vi "Send Message.vi"(6 "Reply to...":refnum<class "Send.lvclass">, 8 "error in (no error)":errorcluster, 10 "Message":refnum<class "MSG.lvclass">, 11 "MSR Parent in":refnum<class "Send.lvclass">) -> (0 "error out":errorcluster, 3 "MSR Parent out":refnum<class "Send.lvclass">)   [LabVIEW 2011, in "Messenging.lvlib" / "Send.lvclass"]
uses:
  Send.lvclass
  TextVarientMessage/MSG.lvclass
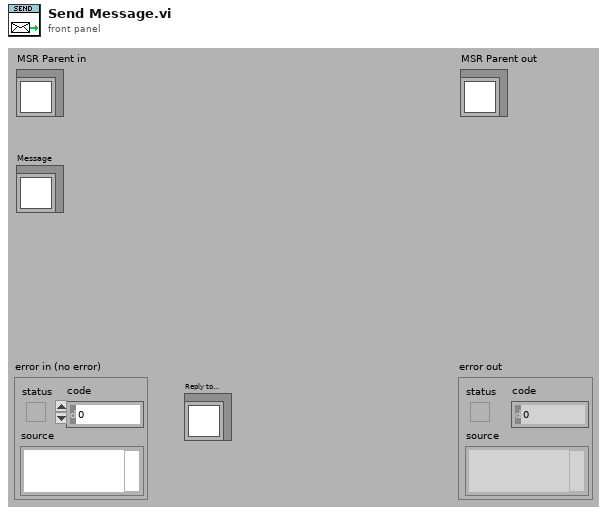
[diagram p1: front panel]
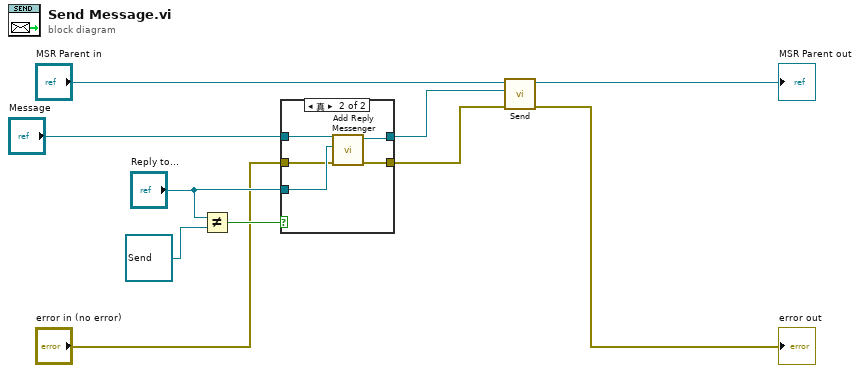
[diagram p0: block diagram]
diagram:
  n1 = Not Equal?(x="Reply to...", y=refnum<class "Send.lvclass"> refnum) -> (x != y?=w4:bool)
  n2 = case shown="真" w4 {
    tunnel: "Message" -> [w11 w17]
    tunnel: "Reply to..." -> [_ w16]
    tunnel: "error in (no error)" -> [w12 w15]
    tunnel: [w12 w14] -> w2
    tunnel: [w11 w13] -> w1
    frame False {
    }
    frame True {
      n3 = call "Add Reply Messenger.vi"("error in (no error)"=w15, "Reply to..."=w16, "Message"=w17) -> ("error out"=w14:errorcluster, "Message"=w13:refnum<class "MSG.lvclass">)  [unwired: 7 out]
    }
  }
  n4 = call-dynamic "Send.vi"("error in (no error)"=w2, "Message"=w1, "MSR Parent in"="MSR Parent in") -> ("error out"=→"error out":errorcluster, "MSR Parent out"=→"MSR Parent out":refnum<class "Send.lvclass">)  [unwired: 7 out]
